vi "setUp.vi"(8 "error in (no error)":errorcluster, 11 "reference in":refnum<class "Logging Loopback.lvclass">) -> (0 "error out":errorcluster, 3 "reference out":refnum<class "Logging Loopback.lvclass">)   [LabVIEW 2020, in "Logging Loopback.lvclass"]
doc: "setUp runs prior to the test method during test execution. Use this method to initialize any object data required by your tests."
uses:
  Logging Loopback.lvclass
  C:/Program Files (x86)/National Instruments/LabVIEW 2020/vi.lib/addons/_JKI Toolkits/VI Tester/TestCase.llb/TestCase.lvclass
  Logging Loopback.lvclass/Logging Loopback.ctl
  <vilib>/addons/_JKI Toolkits/VI Tester/TestCase.llb/TestCase.lvclass
  niveristand-custom-device-testing-tools/VeriStandTestUtilities/VeriStandTestUtilities.lvlib
  <vilib>/WebDAVClient/NI_WebDAV.lvlib
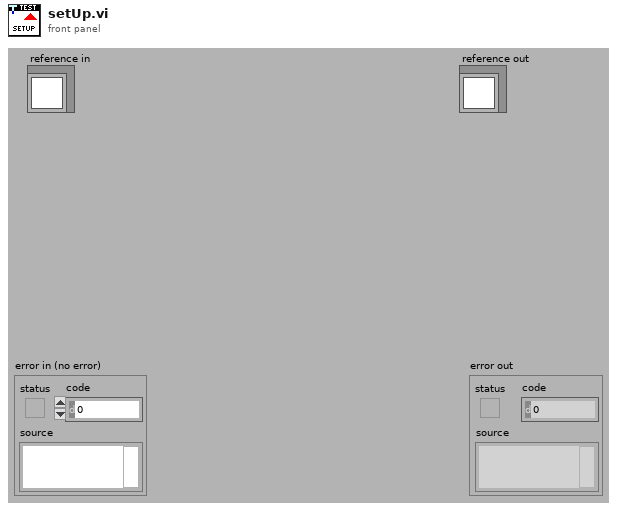
[diagram p1: front panel]
types:
  T1 = typedef "Custom Device API.lvlib/Custom Device Item Ref.ctl" = u64
  T2 = typedef "NI_WebDAV.lvlib/SessionHandle.ctl" = refnum<k1>
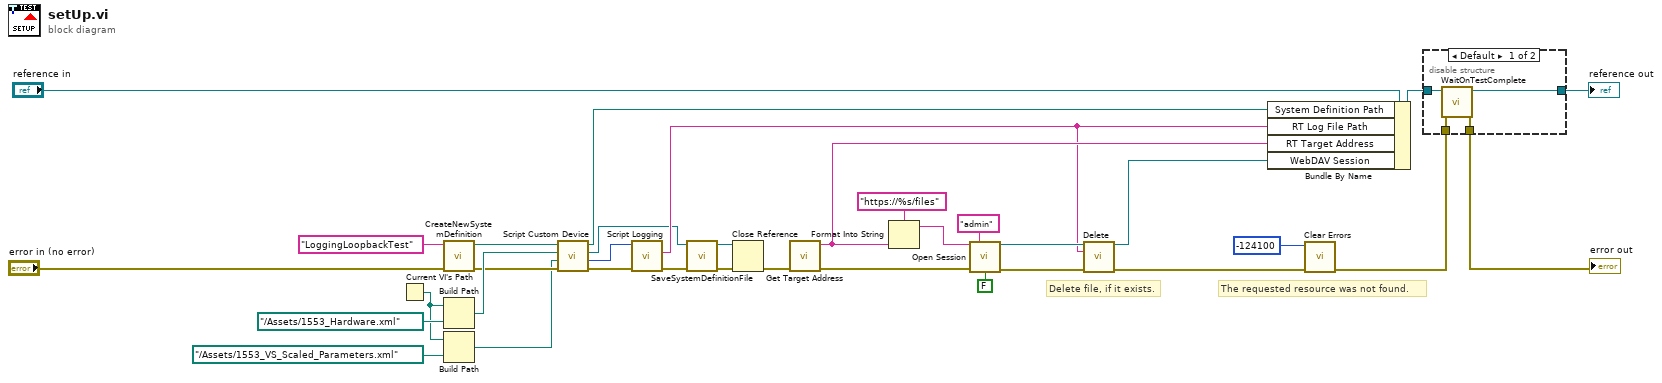
[diagram p0: block diagram]
diagram:
  # "Delete file, if it exists."
  # "The requested resource was not found."
  n1 = Current VI's Path() -> (path=w1:path)
  n2 = call "CreateNewSystemDefinition.vi"("error in"="error in (no error)", "System Definition Name"="LoggingLoopbackTest" ("Channel")) -> ("error out"=w10:errorcluster, "System Definition Path"=w9:path)  [unwired: 8 in]
  n3 = Build Path(base path=w1, name or relative path=path "../Assets/1553_Hardware.xml" ("Hardware File Path")) -> (appended path=w14:path)
  n4 = Build Path(base path=w1, name or relative path=path "../Assets/1553_VS_Scaled_Parameters.xml" ("Hardware File Path")) -> (appended path=w2:path)
  n5 = call "Script Custom Device.vi"("error in"=w10, "parameters configuration file path"=w2, "hardware configuration file path"=w14, "system definition path in"=w9) -> ("error out"=w7:errorcluster, "Ballard MIL-STD 1553 custom device out"=w6:T1, "System Definition"=w8:refnum<k24>, "system definition path out"=w17:path)  [unwired: 4 in]
  n6 = call "Script Logging.vi"("error in (no error)"=w7, "Ballard MIL-STD 1553 custom device in"=w6) -> ("error out"=w5:errorcluster, "RT log file path"=w21:string)  [unwired: 7 in, 1 out]
  n7 = call "SaveSystemDefinitionFile.vi"("error in (no error)"=w5, "System Definition Reference in"=w8) -> ("error out"=w4:errorcluster, "System Definition Reference out"=w3:refnum<k24>)  [unwired: 8 in]
  n8 = Close Reference(reference=w3, error in (no error)=w4) -> (error out=w29:errorcluster)
  n9 = call "Get Target Address.vi"("error in (no error)"=w29) -> ("error out"=w23:errorcluster, "target address"=w22:string)  [unwired: 9 in]
  n10 = Format Into String(format string="https://%s/files" ("host uri prefix"), w22) -> (resulting string=w24:string)  [unwired: 2 in, 1 out]
  n11 = call <vilib>:"Open Session.vi"("host uri prefix"=w24, "username"="admin", "error in (no error)"=w23, "verify server?"=FALSE) -> ("session handle out"=w28:T2, "error out"=w27:errorcluster)  [unwired: 10 in]
  n12 = call <vilib>:"Delete.vi"("session handle"=w28, "relative uri"=w21, "error in (no error)"=w27) -> ("session handle out"=w15:T2, "error out"=w19:errorcluster)  [unwired: 11 in]
  n13 = Bundle By Name(cluster="reference in", "System Definition Path"=w17, "RT Log File Path"=w21, "RT Target Address"=w22, "WebDAV Session"=w15) -> (w30:refnum<class "Logging Loopback.lvclass">)
  n14 = call <vilib>:"Clear Errors.vi"("error in (no error)"=w19, "specific error code to clear (0: all)"=-124100) -> ("error out"=w16:errorcluster)  [unwired: 4 in, 1 out]
  n15 = disable-structure shown="Default" {
    disable-tunnel: w16 -> [w38 w39]
    disable-tunnel: [w37 w39] -> w34
    disable-tunnel: [w36 w40] -> w32
    disable-tunnel: w30 -> [w35 w40]
    frame condition #0 (active) {
      n16 = call <vilib>:"WaitOnTestComplete.vi"("error in (no error)"=w38, "TestCase in"=w35) -> ("error out"=w37:errorcluster, "TestCase out"=w36:refnum<class "Logging Loopback.lvclass">)  [unwired: 8 in]
    }
    frame condition #1 {
    }
  }
  "error out" <- w34
  "reference out" <- w32
